vi "Configure ARC.vi"(0 "VISA resource name":refnum<visa-resource-name>, 5 "ARC Input":string="0", 7 "Configuration Query":bool=TRUE, 11 "error in (no error)":errorcluster) -> (4 "VISA resource name out":refnum<visa-resource-name>, 6 "Query Output":string="\r\n", 8 "Error Message":string, 10 "Error Code":i32, 15 "error out":errorcluster)   [LabVIEW 2010, in "VITREK V7X.lvlib"]
doc: "Configures or Query the <b>ARC</b> current limit (0 = disabled).\n\n<b>Note:</b> please refer to the instrument manual for the <b>ARC</b> current limit specification."
uses:
  VITREK V7X.lvlib
panel:
  # "Yes\n\nNo"
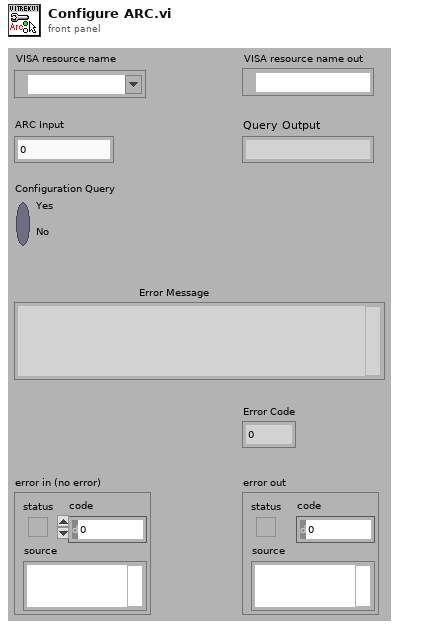
[diagram p1: front panel]
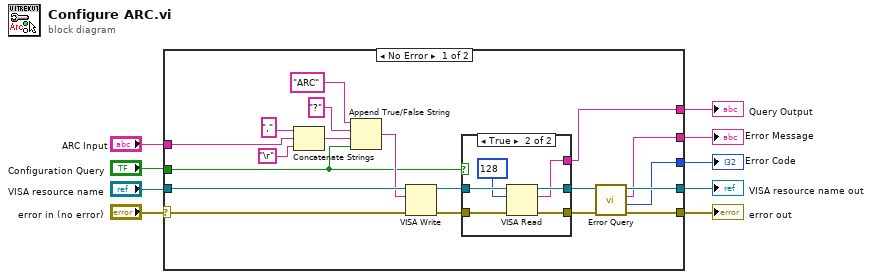
[diagram p0: block diagram]
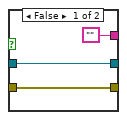
[diagram p2: hidden frame]
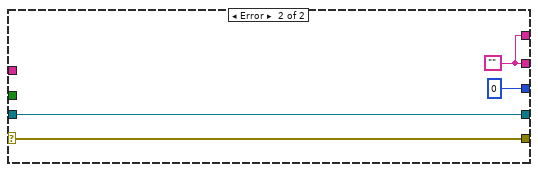
[diagram p3: hidden frame]
diagram:
  n1 = case shown="No Error" "error in (no error)" {
    selector: "error in (no error)" -> [w17 w40]
    tunnel: "VISA resource name" -> [w28 w41]
    tunnel: "Configuration Query" -> [w24 _]
    tunnel: [w22 w39] -> w7
    tunnel: [w19 w41] -> w6
    tunnel: [w18 w40] -> w5
    tunnel: "ARC Input" -> [w13 _]
    tunnel: [w12 0 ("Error Code")] -> w2
    tunnel: [w11 w39] -> w1
    frame No Error {
      n2 = Concatenate Strings(",", w13, "\r") -> (w14:string)
      n3 = Append True/False String(1:w24, 2:w14, 3:"?", 4:"ARC" ("command")) -> (0:w26:string)
      n4 = VISA Write(VISA resource name=w28, write buffer=w26, error in (no error)=w17) -> (VISA resource name out=w25:refnum<visa-resource-name>, error out=w23:errorcluster)  [unwired: 1 out]
      n5 = case shown="True" w24 {
        tunnel: w25 -> [w31 w35]
        tunnel: [w31 w33] -> w21
        tunnel: w23 -> [w30 w36]
        tunnel: [w30 w37] -> w20
        tunnel: ["" w32] -> w22
        frame False {
        }
        frame True {
          n6 = VISA Read(VISA resource name=w35, byte count=u32 128, error in (no error)=w36) -> (VISA resource name out=w33:refnum<visa-resource-name>, read buffer=w32:string, error out=w37:errorcluster)  [unwired: 1 out]
        }
      }
      n7 = call "Error Query.vi"("error in (no error)"=w20, "VISA resource name"=w21) -> ("error out"=w18:errorcluster, "Error Code"=w12:i32, "Error Message"=w11:string, "VISA resource name out"=w19:refnum<visa-resource-name>)  [unwired: 6 in]
    }
    frame Error {
      w39 = ""
    }
  }
  "VISA resource name out" <- w6
  "error out" <- w5
  "Query Output" <- w7
  "Error Code" <- w2
  "Error Message" <- w1
